vi "SMBUS Read Byte Protocol.vi"(5 "WithPEC":u8, 6 "pData":u8, 7 "CommandCode":u8, 9 "SlaveAddr":i16, 10 "IICIndex":i32, 11 "DevHandle":i32) -> (3 "function return":i32, 4 "pData out":u8)   [LabVIEW 2010, in "usb2iic.lvlib"]
doc: "int WINAPI SMBUS_ReadByteProtocol(int DevHandle,int IICIndex,short SlaveAddr,unsigned char CommandCode, unsigned char *pData,unsigned char WithPEC);"
uses:
  usb2iic.lvlib
  USB2XXX.dll
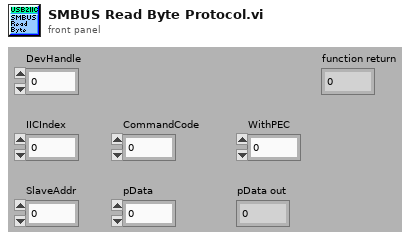
[diagram p1: front panel]
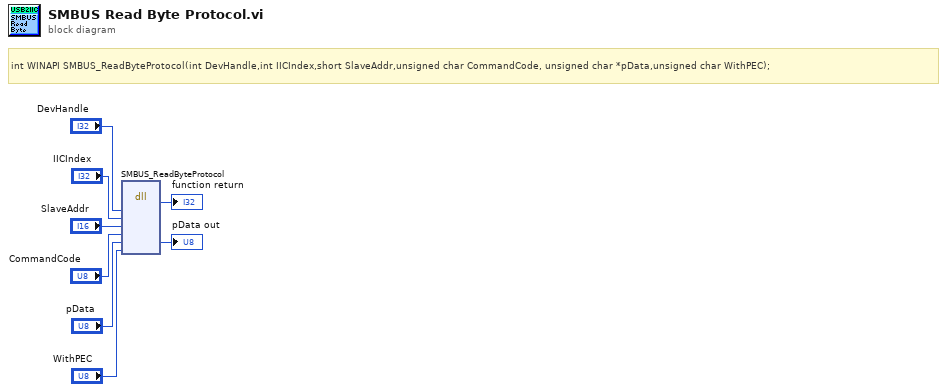
[diagram p0: block diagram]
diagram:
  # "int WINAPI SMBUS_ReadByteProtocol(int DevHandle,int IICIndex,short SlaveAddr,unsigned char CommandCode, unsigned char *pData,unsigned char WithPEC);"
  n1 = dll-call lib="G:/OtherWork/USB2XXX_Example/trunk/Labview/PublicFiles/usb2iic/USB2XXX.*" fn="SMBUS_ReadByteProtocol"("DevHandle"="DevHandle", "IICIndex"="IICIndex", "SlaveAddr"="SlaveAddr", "CommandCode"="CommandCode", "pData"="pData", "WithPEC"="WithPEC") -> (→"function return":i32, "pData"=→"pData out":u8)  [unwired: 8 in, 2 out]
